vi "UI.vi"() -> ()   [LabVIEW 2017]
panel:
  out "Fast":bool
  out "Slow":bool
  out "Stop":bool
  out "Start":bool
  out "Temperature":dbl(slide) scale=0.0..100.0
  in  "Enable Motor":bool
  out "Output":sgl
  in  "Reset":bool
  in  "Strain":sgl
  out "Chart":sgl format="%#.10g"
  in  "Slider":sgl(slide) scale=0.0..10.0
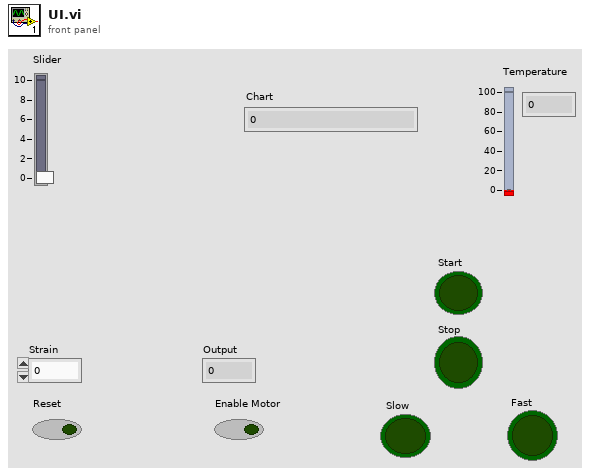
[diagram p1: front panel]
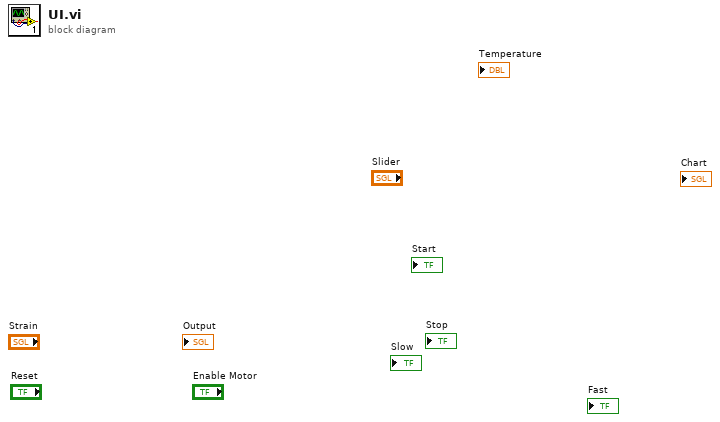
[diagram p0: block diagram]
diagram:
